vi "Text Editor Path--constant.vi"() -> (3 "Path":path)   [LabVIEW 2025]
doc: "Path to text editor application."
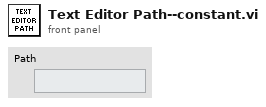
[diagram p1: front panel]
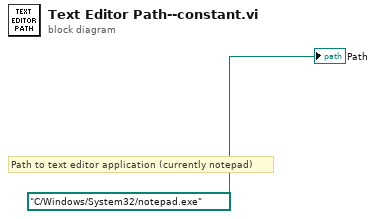
[diagram p0: block diagram]
diagram:
  # "Path to text editor application (currently notepad)"
  "Path" <- path "C:/Windows/System32/notepad.exe" ("Exe Path")
